vi "Sample Transfer Query Cold Block TC.vi"(7 "Container":T1, 8 "error in (no error)":errorcluster, 10 "Switch OFF when Done (True)":bool=TRUE, 11 "cRIO-CO2 in":refnum<class "cRIO-CO2.lvclass">) -> (0 "error out":errorcluster, 3 "cRIO-CO2 out":refnum<class "cRIO-CO2.lvclass">, 4 "Warmed up?":bool)   [LabVIEW 2015, in "cRIO-Carbondioxide.lvlib" / "cRIO-CO2.lvlib" / "cRIO-CO2.lvclass"]
uses:
  cRIO-CO2.lvclass
  Controls/Sample Transfer Container Enumerator.ctl
  Blowers Heaters Enumerator.ctl
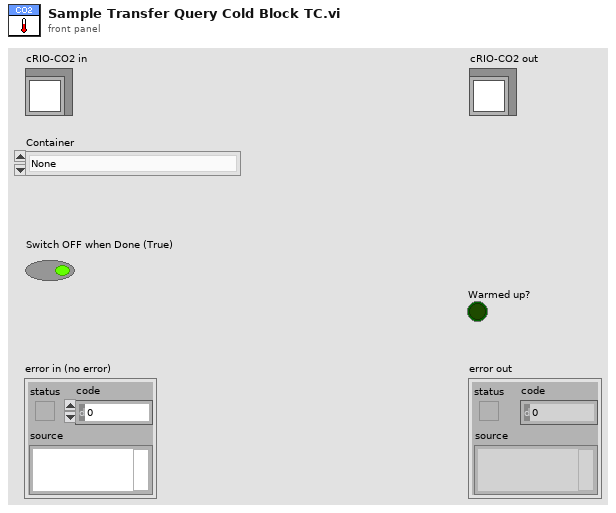
[diagram p1: front panel]
types:
  T1 = typedef "Sample Transfer Container Enumerator.ctl" = enum16{"None", "Sample 1", "Sample 2", "Sample 3", "Sample 4", "Sample 5", "Storage 01", "Storage 02", "Storage 03", "Storage 04", "Storage 05", "Storage 06", "Storage 07", "Storage 08", "Storage 09", "Storage 10", "Storage 11", "Storage 12", "Syringe", "Undefined"}
  T2 = typedef "cRIO-Carbondioxide.lvlib/cRIO-CO2.lvlib/cRIO-CO2.lvclass/Blowers Heaters Enumerator.ctl" = enum16{"Tank Blower 1", "Tank Blower 2", "Tank Blower 3", "Tank Blower 4", "Syringe Blower", "Syringe Heater", "Piston Heater", "Undefined"}
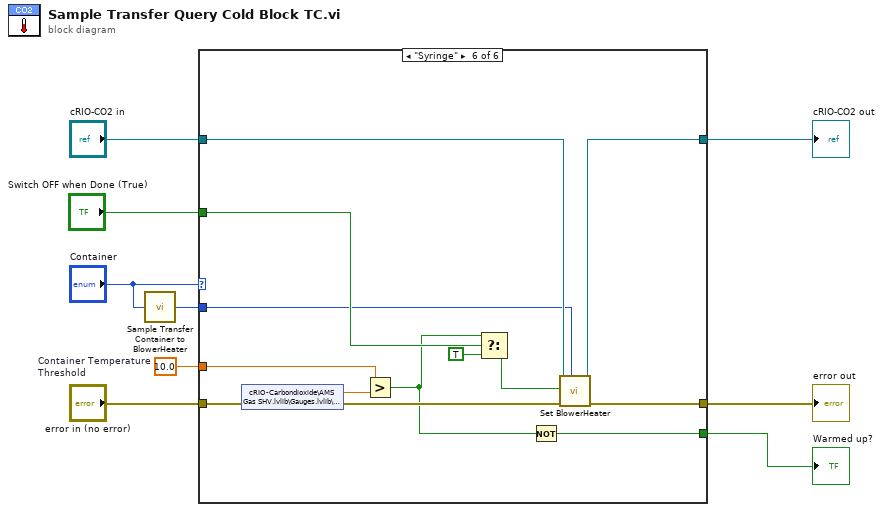
[diagram p0: block diagram]
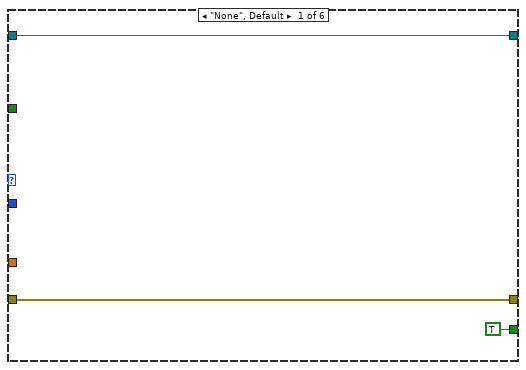
[diagram p2: hidden frame]
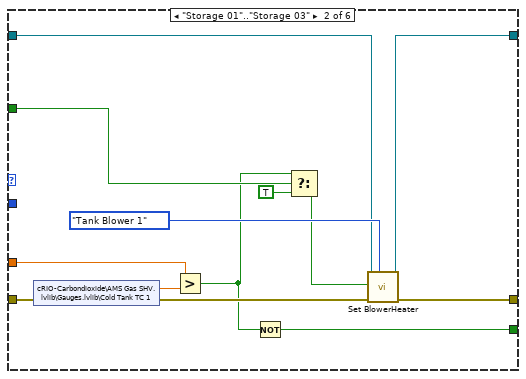
[diagram p3: hidden frame]
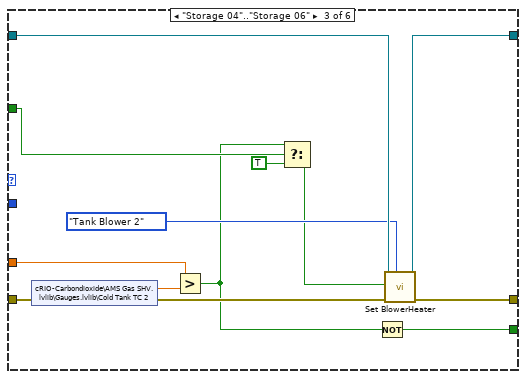
[diagram p4: hidden frame]
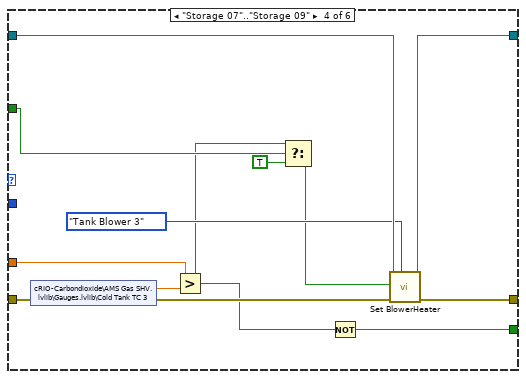
[diagram p5: hidden frame]
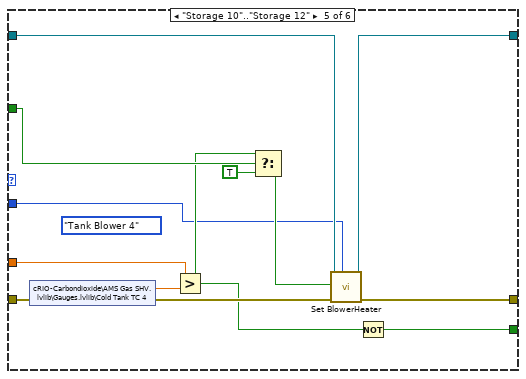
[diagram p6: hidden frame]
diagram:
  w9 = 10.0  # Container Temperature Threshold
  n1 = call "Sample Transfer Container to BlowerHeater.vi"("Container"="Container") -> ("Blower/Heater"=w1:T2)  [unwired: 4 in]
  n2 = case shown="\"Syringe\"" "Container" {
    tunnel: "error in (no error)" -> [w11 w25 w37 w50 w63 w76]
    tunnel: "cRIO-CO2 in" -> [w12 w20 w34 w46 w59 w73]
    tunnel: [w12 w19 w33 w45 w58 w72] -> w5
    tunnel: [w11 w18 w31 w47 w60 w71] -> w7
    tunnel: w9 -> [_ w23 w38 w51 w64 w77]
    tunnel: [TRUE w17 w30 w43 w57 w70] -> w4
    tunnel: "Switch OFF when Done (True)" -> [_ w15 w28 w41 w55 w69]
    tunnel: w1 -> [_ _ _ _ w52 w65]
    frame "None", Default {
    }
    frame "Storage 01".."Storage 03" {
      n3 = shared-variable "cRIO-Carbondioxide\\AMS Gas SHV.lvlib\\Gauges.lvlib\\Cold Tank TC 1"(error in=w25) -> (w24:dbl, error out=w22:errorcluster)
      n4 = Greater?(x=w23, y=w24) -> (0:w14:bool)
      n5 = Not(x=w14) -> (.not. x?=w17:bool)
      n6 = Select(t=w14, s=w15, f=TRUE) -> (s? t:f=w13:bool)
      n7 = call "Set BlowerHeater.vi"("Blower/Heater"=Blowers_Heaters_Enumerator."Tank Blower 1" ("Blower"), "error in (no error)"=w22, "ON/OFF (OFF)"=w13, "cRIO-CO2 in"=w20) -> ("error out"=w18:errorcluster, "cRIO-CO2 out"=w19:refnum<class "cRIO-CO2.lvclass">)  [unwired: 6 in]
    }
    frame "Storage 04".."Storage 06" {
      n8 = shared-variable "cRIO-Carbondioxide\\AMS Gas SHV.lvlib\\Gauges.lvlib\\Cold Tank TC 2"(error in=w37) -> (w36:dbl, error out=w35:errorcluster)
      n9 = Greater?(x=w38, y=w36) -> (0:w27:bool)
      n10 = Select(t=w27, s=w28, f=TRUE) -> (s? t:f=w26:bool)
      n11 = Not(x=w27) -> (.not. x?=w30:bool)
      n12 = call "Set BlowerHeater.vi"("Blower/Heater"=Blowers_Heaters_Enumerator."Tank Blower 2" ("Blower"), "error in (no error)"=w35, "ON/OFF (OFF)"=w26, "cRIO-CO2 in"=w34) -> ("error out"=w31:errorcluster, "cRIO-CO2 out"=w33:refnum<class "cRIO-CO2.lvclass">)  [unwired: 6 in]
    }
    frame "Storage 07".."Storage 09" {
      n13 = shared-variable "cRIO-Carbondioxide\\AMS Gas SHV.lvlib\\Gauges.lvlib\\Cold Tank TC 3"(error in=w50) -> (w49:dbl, error out=w48:errorcluster)
      n14 = Greater?(x=w51, y=w49) -> (0:w40:bool)
      n15 = Select(t=w40, s=w41, f=TRUE) -> (s? t:f=w39:bool)
      n16 = Not(x=w40) -> (.not. x?=w43:bool)
      n17 = call "Set BlowerHeater.vi"("Blower/Heater"=Blowers_Heaters_Enumerator."Tank Blower 3" ("Blower"), "error in (no error)"=w48, "ON/OFF (OFF)"=w39, "cRIO-CO2 in"=w46) -> ("error out"=w47:errorcluster, "cRIO-CO2 out"=w45:refnum<class "cRIO-CO2.lvclass">)  [unwired: 6 in]
    }
    frame "Storage 10".."Storage 12" {
      (unwired) Blowers_Heaters_Enumerator."Tank Blower 4" ("Blower")
      n18 = shared-variable "cRIO-Carbondioxide\\AMS Gas SHV.lvlib\\Gauges.lvlib\\Cold Tank TC 4"(error in=w63) -> (w62:dbl, error out=w61:errorcluster)
      n19 = Greater?(x=w64, y=w62) -> (0:w54:bool)
      n20 = Select(t=w54, s=w55, f=TRUE) -> (s? t:f=w53:bool)
      n21 = call "Set BlowerHeater.vi"("Blower/Heater"=w52, "error in (no error)"=w61, "ON/OFF (OFF)"=w53, "cRIO-CO2 in"=w59) -> ("error out"=w60:errorcluster, "cRIO-CO2 out"=w58:refnum<class "cRIO-CO2.lvclass">)  [unwired: 6 in]
      n22 = Not(x=w54) -> (.not. x?=w57:bool)
    }
    frame "Syringe" {
      n23 = shared-variable "cRIO-Carbondioxide\\AMS Gas SHV.lvlib\\Gauges.lvlib\\Syringe TC"(error in=w76) -> (w75:dbl, error out=w74:errorcluster)
      n24 = Greater?(x=w77, y=w75) -> (0:w67:bool)
      n25 = Select(t=w67, s=w69, f=TRUE) -> (s? t:f=w66:bool)
      n26 = Not(x=w67) -> (.not. x?=w70:bool)
      n27 = call "Set BlowerHeater.vi"("Blower/Heater"=w65, "error in (no error)"=w74, "ON/OFF (OFF)"=w66, "cRIO-CO2 in"=w73) -> ("error out"=w71:errorcluster, "cRIO-CO2 out"=w72:refnum<class "cRIO-CO2.lvclass">)  [unwired: 6 in]
    }
  }
  "error out" <- w7
  "cRIO-CO2 out" <- w5
  "Warmed up?" <- w4
